vi "Process CCON_CPOS.vi"(11 "FHPP in":refnum<class "FHPP.lvclass">) -> (2 "Desired Operating Mode":T1, 3 "FHPP out":refnum<class "FHPP.lvclass">)   [LabVIEW 2022 SP3, in "FHPP.lvclass"]
uses:
  FHPP.lvclass
  FHPP.lvclass/FHPP.ctl
  TypeDefs/Operating Mode.ctl
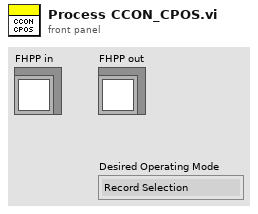
[diagram p1: front panel]
types:
  T1 = typedef "FHPP.lvclass/Operating Mode.ctl" = enum16{"Record Selection", "Direct Mode", "Reserved 1", "Reserved 2"}
  T2 = typedef "FHPP.lvclass/CCON.ctl" = cluster{"Enabled Drive":bool, "Stop":bool, "Open Brake":bool, "Reset Fault":bool, "Reserved":bool, "Lock Software Access":bool, "Operating Mode":T1}
  T3 = typedef "FHPP.lvclass/CPOS.ctl" = cluster{"Halt":bool, "Start":bool, "Start Homing":bool, "Jog Positive":bool, "Jog Negative":bool, "Teach Actual Value":bool, "Clear Remaining Pos":bool, "Reserved":bool}
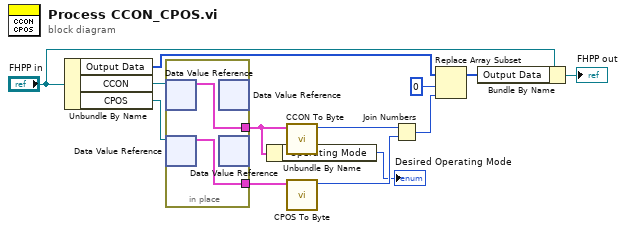
[diagram p0: block diagram]
diagram:
  n1 = Unbundle By Name("FHPP in") -> ("Output Data"=w7:u16[], "CCON"=w5:refnum<data-value>, "CPOS"=w6:refnum<data-value>)
  n2 = in-place {
    in-place-border: [w15] -> w3
    in-place-border: [w14] -> w2
    n3 = in-place-dvr #1(w5) -> (w14:T2)  [unwired: 1 out]
    n4 = in-place-dvr #2(w6) -> (w15:T3)  [unwired: 1 out]
    n5 = in-place-dvr #1() -> ()  [unwired: 1 in, 2 out]
    n6 = in-place-dvr #2() -> ()  [unwired: 1 in, 2 out]
  }
  n7 = Unbundle By Name(w2) -> ("Operating Mode"=→"Desired Operating Mode":T1)
  n8 = call "CCON To Byte.vi"("CCON"=w2) -> ("Numeric"=w9:u8)  [unwired: 10 in]
  n9 = call "CPOS To Byte.vi"("CPOS"=w3) -> ("Numeric"=w10:u8)  [unwired: 10 in]
  n10 = Join Numbers(hi=w9, lo=w10) -> ((hi.lo)=w11:u16)
  n11 = Replace Array Subset(array=w7, new element=w11, index=0) -> (w12:u16[])
  n12 = Bundle By Name(cluster="FHPP in", "Output Data"=w12) -> (→"FHPP out":refnum<class "FHPP.lvclass">)
